vi "Process.vi"(8 "error in":errorcluster, 11 "Oxford1820 UI in":refnum<class "Instrument UI.Oxford1820.lvclass">) -> (0 "error out":errorcluster, 3 "Oxford1820 UI out":refnum<class "Instrument UI.Oxford1820.lvclass">)   [LabVIEW 2019, in "Instrument UI.Oxford1820.lvclass"]
doc: "---------------------------------------------------------------\nJKI State Machine Objects™\nhttp://jki.net/state-machine-objects/\nCopyright (C) 2005-2015, JKI <info@jki.net>\nALL RIGHTS RESERVEDJKI State Machine Objects (SMO) 1.0.0.5\nJKI - JKI\nCopyright (c) 2016, JKI"
uses:
  Instrument UI.Oxford1820.lvclass
  C:/Program Files/National Instruments/LabVIEW 2019/vi.lib/JKI/JKI SMO/SMO/SMO.lvclass
  C:/Program Files/National Instruments/LabVIEW 2019/user.lib/LevyLab/Instrument Framework/Instrument UI/Instrument UI.lvclass
  C:/Program Files/National Instruments/LabVIEW 2019/vi.lib/JKI/JKI SMO/SMO.UI/SMO.UI.lvclass
  <instrlib>/Mercury iXX/Public/Libraries/Magnet/Controls/Switch Heater.ctl
  Instrument.Oxford1820/Typedefs/getAll.ctl
  Instrument.Oxford1820/Instrument.Oxford1820.lvclass
  C:/Program Files/National Instruments/LabVIEW 2019/user.lib/LevyLab/Instrument Framework/Instrument/Instrument.lvclass
  <userlib>/LevyLab/Instrument Framework/Instrument UI/Instrument UI.lvclass/Instrument UI.ctl
  Instrument.Oxford1820/Instrument.Oxford1820.lvclass/Instrument.Oxford1820.ctl
  <vilib>/JKI/JKI SMO/SMO/SMO.lvclass/SMO.ctl
  <userlib>/LevyLab/Instrument Framework/Instrument/Typedefs/Client Type--Enum.ctl
  <userlib>/LevyLab/Instrument Framework/Instrument/Instrument.lvclass/Instrument.ctl
  Instrument.Oxford1820/Typedefs/Fill Mode-Combo.ctl
  <vilib>/JKI/JKI SMO/SMO/Private/ReftoDVR--SMO.vi
  <userlib>/LevyLab/Instrument Framework/Instrument/Instrument.lvclass
  <userlib>/LevyLab/Instrument Framework/Instrument UI/Instrument UI.lvclass
  <vilib>/JKI/JKI SMO/SMO/SMO.lvclass
  <vilib>/JKI/JKI SMO/SMO.UI/SMO.UI.lvclass
  <instrlib>/Mercury iXX/Public/Libraries/Magnet.lvlib
panel:
  in  "Clamp":bool
  in  "Open Target":dbl=100.0 format="%.1f (%%)"
  out "System Time (HH:MM:SS)":dbl=165.3592643737793 format="%<%I:%M:%S %p>T"
  out "LPF on":dbl format="%<%H:%M:%S>t"
  out "PS Heat on (HH:MM:SS)":dbl format="%<%H:%M:%S%1u>t"
  out "ETA":dbl=3660699600.0 format="%<%I:%M:%S %p %m/%d/%Y>T"
  out "version":string="v20/10/28"
  out "Level Graph":cluster{timestamp[], dbl[]}[](graph)
  out "N2 LEVEL":dbl format="%.0f %"
  in  "Window Maximize":bool
  in  "Window Minimize":bool
  out "Magnet Status 3":string="Status: Clamped"
  out "Voltage Meter":dbl(knob) caption="Voltage (V)" scale=-10.0..10.0
  out "Current Meter":dbl(knob) caption="Voltage (V)" scale=-180.0..180.0
  out "Magnet Field Meter":dbl(knob) caption="Voltage (V)" scale=-20.0..20.0
  in  "Hold":bool
  in  "To Set":bool
  in  "Send To IPS":bool
  out "PSU Field":dbl format="%#.5f T"
  in  "Target Field (T)":dbl caption="Field" format="%.2f"
  out "Target Field (T)":dbl caption="Field" format="%.2f T"
  in  "Target Rate (T/min)":dbl=0.1 caption="Rate" min=0.0 max=1.0 format="%.2f"
  out "Target Rate (T/min)":dbl caption="Rate" format="%.2f T/min"
  out "Field":dbl format="%.5f T"
  out "He LEVEL":dbl format="%.0f %"
  in  "PS Heat":bool
  in  "To Zero":bool
  out "N2 LVL":dbl format="%.1f (%%)"
  out "He LVL Chart":dbl(slide)=52.0833 scale=0.0..100.0
  out "N2 LVL Chart":dbl(slide)=61.3025 scale=0.0..100.0
  out "He LVL":dbl format="%.1f (%%)"
  in  "Fast/Slow Fill":bool
  in  "Open Needle Valve":bool
  in  "Close Needle Valve":bool
  in  "LPF Power":bool
  out "Needle Valve":dbl format="%.1f (%%)"
  out "Pressure":dbl format="%_5f mB"
  out "Magnet T":dbl format="%_2f K"
  out "Magnet R":dbl format="%_3f ohms"
  out "Voltage":dbl format="%.5f V"
  out "Current":dbl format="%.5f A"
  out "Magnet Status 2":string="Status: Clamped"
  # "Actions"
  # "Targets"
  # "Status"
  # "LPF"
  # "Needle Valve"
  # "IPS"
  # "PS Switch"
  # "Level"
  # "Level Graph"
  # "Rates"
  # "Slow Rates\nCurrent Range (A)     Field Range (T)  Rate (T/min)\n0       -- 100        0    -- 11.5     0.91\n100     -- 150        11.5 -- 17.2     0.23\n150     -- 155.467    17.2 -- 18       0.11\n155.567 -- 172.471    18   -- 20       0.11\nFast Rates\nCurrent Range (A)     Field Range (T)  Rate (T/min)\n0       -- 155.467    0    -- 18       1.0\n155.567 -- 172.471    18   -- 20       0.25"
  # "Helium"
  # "Nitrogen"
  # "Slow Rates\nCurrent Range (A)     Field Range (T)   Rate (T/min)\n0       -- 100        0    -- 11.5      0.91\n100     -- 150        11.5 -- 17.2      0.23\n150     -- 155.467    17.2 -- 18        0.11\n155.567 -- 172.471    18   -- 20        0.11\n\nFast Rates\nCurrent Range (A)     Field Range (T)   Rate (T/min)\n0       -- 155.467    0    -- 18        1.0\n155.567 -- 172.471    18   -- 20        0.25"
  # "SMO UI Template"
  # "For instructions on how to use the JKI State Machine Objects, examples and video tutorials, visit:\nhttp://jki.net/state-machine-objects/\n\nJKI State Machine Objects™\nhttp://jki.net/state-machine-objects/\nCopyright (C) 2005-2015, JKI <info@jki.net>\nALL RIGHTS RESERVED"
  # "Voltage (V)"
  # "Current (A)"
  # "Magnet (T)"
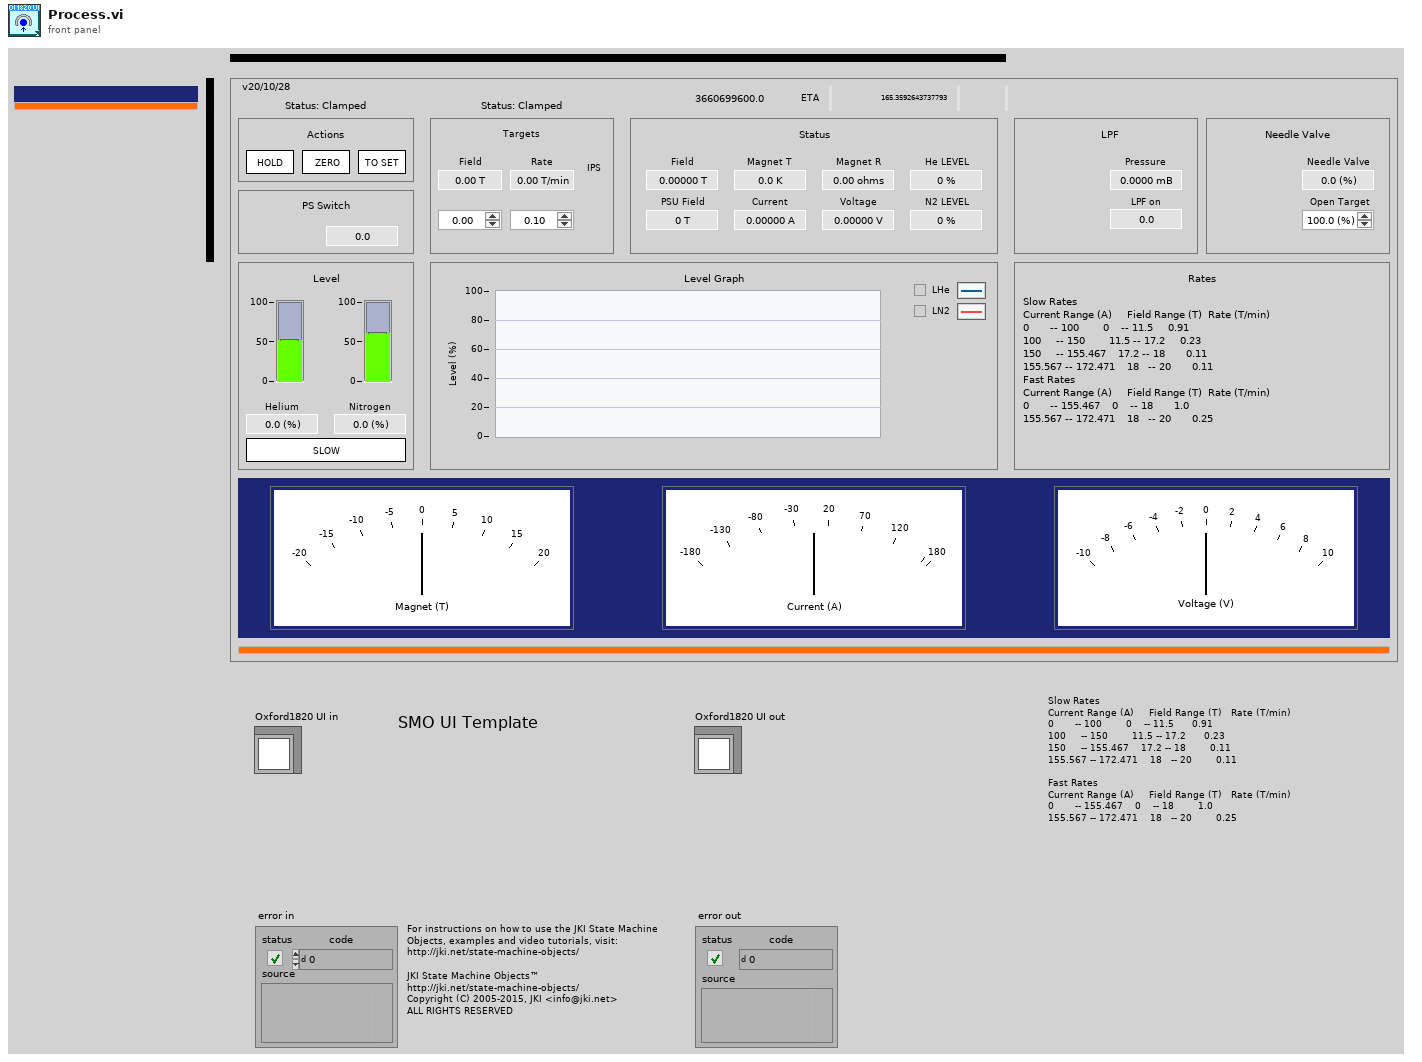
[diagram p1: front panel]
types:
  T1 = typedef "Mercury iXX.lvlib/Magnet.lvlib/Switch Heater.ctl" = string
  T2 = typedef "Instrument.Oxford1820.lvclass/getAll.ctl" = cluster{"1820_IPS_Magnet_Field":dbl, "1820_IPS_PS_Field":dbl, "1820_IPS_Target_Field":dbl, "1820_IPS_Target_Field_Rate":dbl, "1820_IPS_Voltage":dbl, "1820_IPS_Current":dbl, "1820_IPS_Level_N2":dbl, "1820_IPS_Level_He":dbl, "1820_IPS_Magnet_Temperature":dbl, "1820_IPS_Magnet_Temperature_R":dbl, "1820_IPS_M1_Current":dbl, "1820_IPS_M1_Voltage":dbl, "1820_IPS_M2_Current":dbl, "1820_IPS_M2_Voltage":dbl, "1820_IPS_M3_Current":dbl, "1820_IPS_M3_Voltage":dbl, "1820_IPS_Status":string, "1820_IPS_Switch":string, "1820_ITC_Lambda_Temperature":dbl, "1820_ITC_Lambda_Temperature_R":dbl, "1820_ITC_Pressure":dbl, "1820_ITC_Needle_Valve":dbl}
  T3 = enum32{"invalid app kind", "Development System", "Run Time System", "Student Edition", "Embedded LabVIEW", "Evaluation", "Custom"}
  T4 = enum32{"Invalid", "Standard", "Closed", "Hidden", "Minimized", "Maximized"}
  T5 = typedef "Instrument.lvlib/Instrument.lvclass/Client Type--Enum.ctl" = enum16{"Remote", "Local"}
  T6 = typedef "Instrument.Oxford1820.lvclass/Fill Mode-Combo.ctl" = string
  T7 = typedef "RemoteControl.lvlib/RemoteControl.lvclass/Message--Cluster.ctl" = cluster{"Command":string, "Data":variant, "ID":string, "error":errorcluster}
  T8 = cluster{"Core":cluster{"Current VI Reference":refnum<vi>, "Close Panel on Exit?":bool, "error":errorcluster}, "Instrument UI":refnum<class "Instrument UI.Oxford1820.lvclass">, "Instrument":refnum<class "Instrument.Oxford1820.lvclass">, "getAll":T2, "Response":string, "config":variant, "switch time on":timestamp, "switch time off":timestamp, "LPF time":timestamp}
  T9 = typedef "Instrument.Oxford1820.lvclass/PublicEvents--Instrument.Oxford1820.ProcessStatus.ctl" = string
  T10 = cluster{"Current VI Reference":refnum<vi>, "Close Panel on Exit?":bool, "error":errorcluster}
  T11 = typedef "LVRectTypeDef.ctl" = cluster{"Left":i16, "Top":i16, "Right":i16, "Bottom":i16}
  T12 = typedef "SMO.lvclass/Protected Events.ctl" = cluster{"StopProcesses":refnum<user-event>, "AbortProcesses":refnum<user-event>, "Config Changed":refnum<user-event>, "Dependency":refnum<user-event>}
  T13 = typedef "Instrument.lvlib/Instrument.lvclass/PublicEvents--Cluster.ctl" = cluster{"MessageFromProcess":refnum<user-event>}
  T14 = typedef "Instrument.Oxford1820.lvclass/PublicEvents--Cluster.ctl" = cluster{"ProcessStatus":refnum<user-event>}
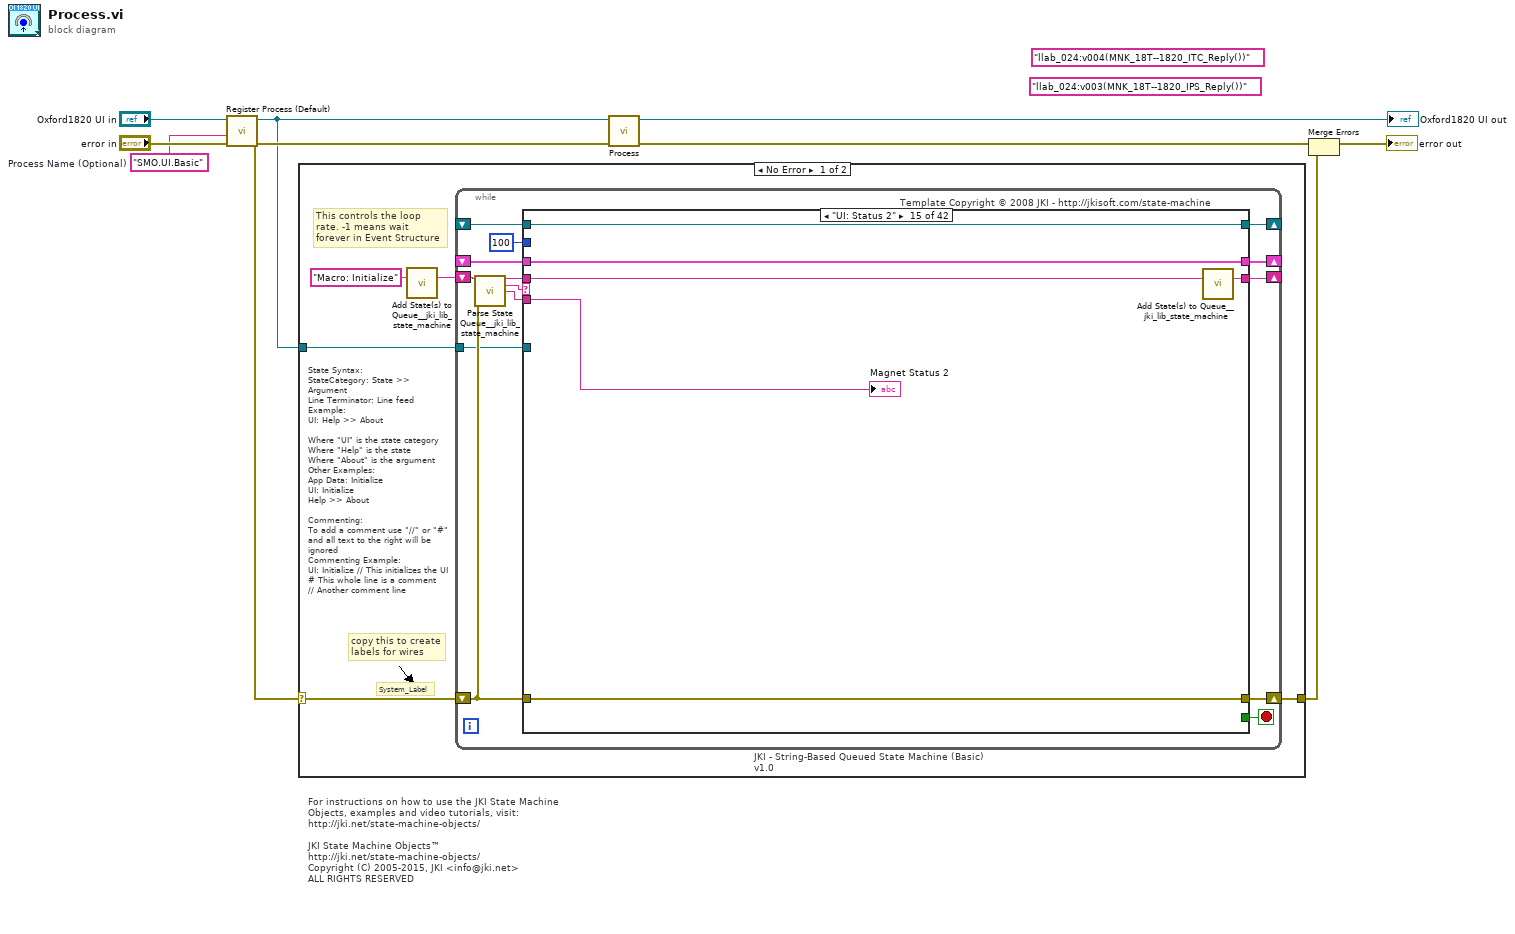
[diagram p0: block diagram]
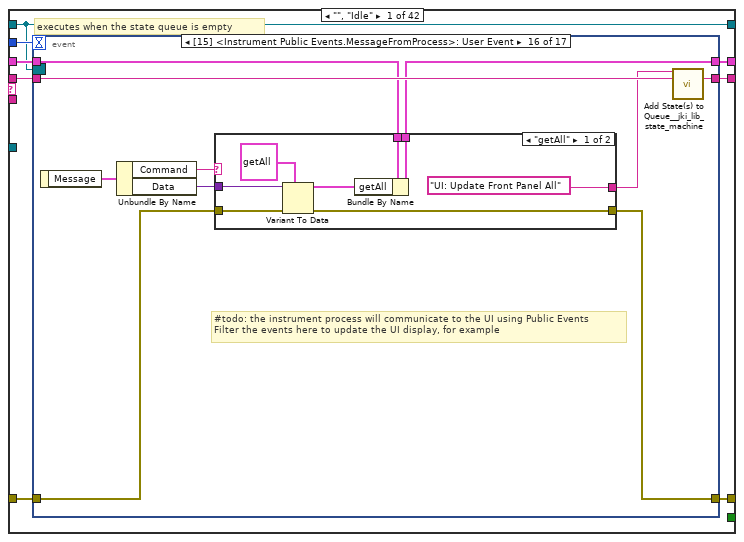
[diagram p2: hidden frame]
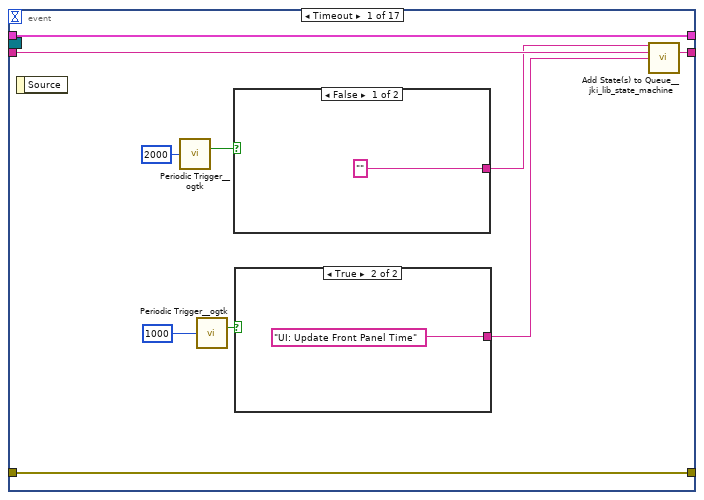
[diagram p3: hidden frame]
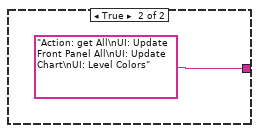
[diagram p4: hidden frame]
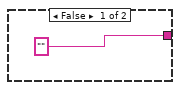
[diagram p5: hidden frame]
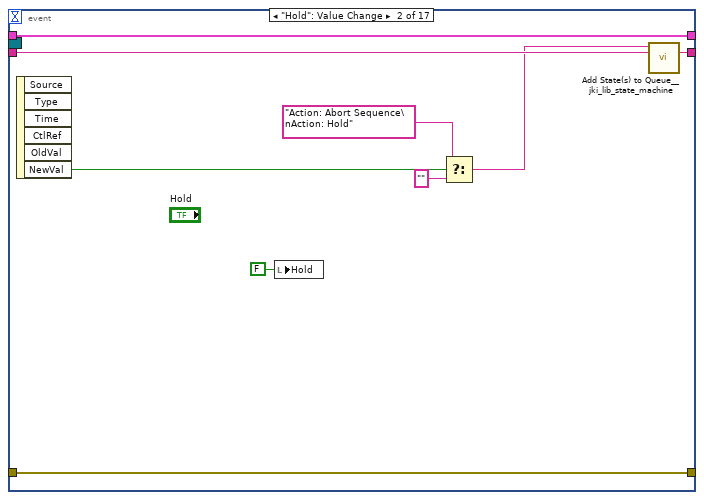
[diagram p6: hidden frame]
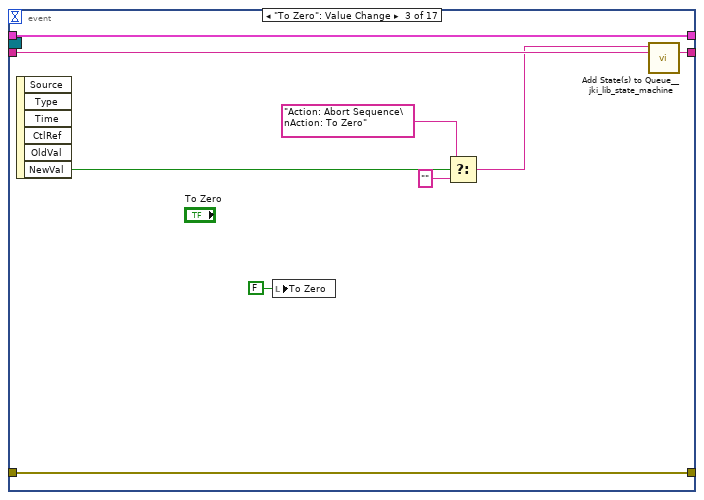
[diagram p7: hidden frame]
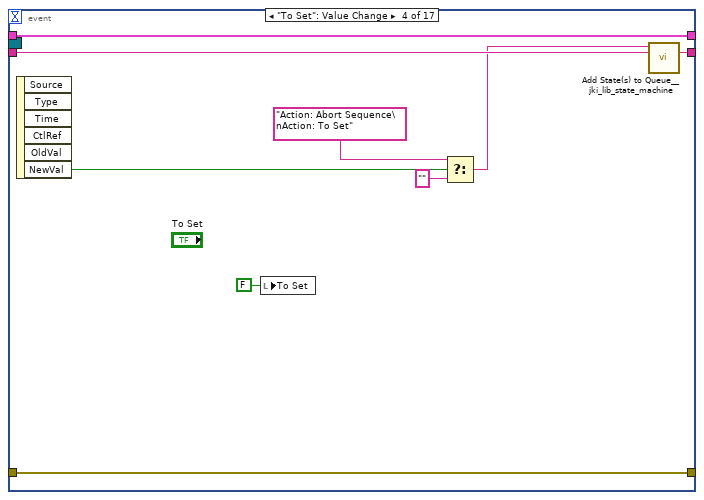
[diagram p8: hidden frame]
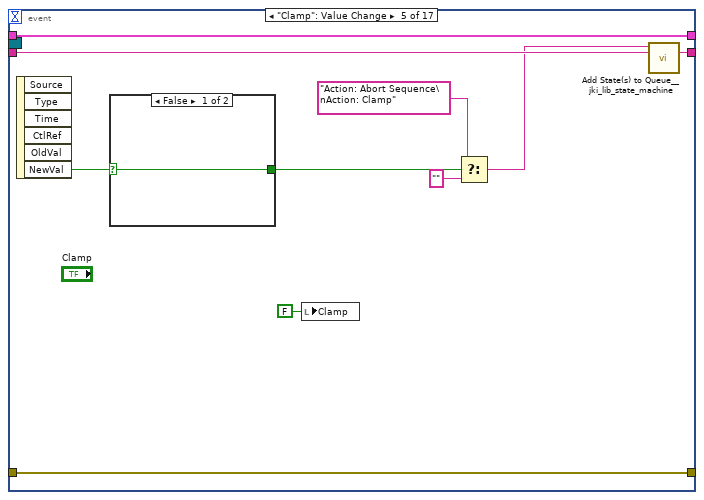
[diagram p9: hidden frame]
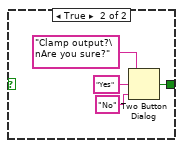
[diagram p10: hidden frame]
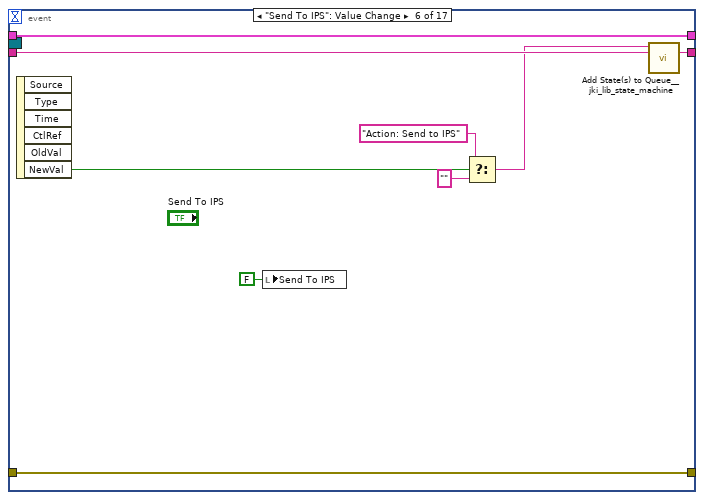
[diagram p11: hidden frame]
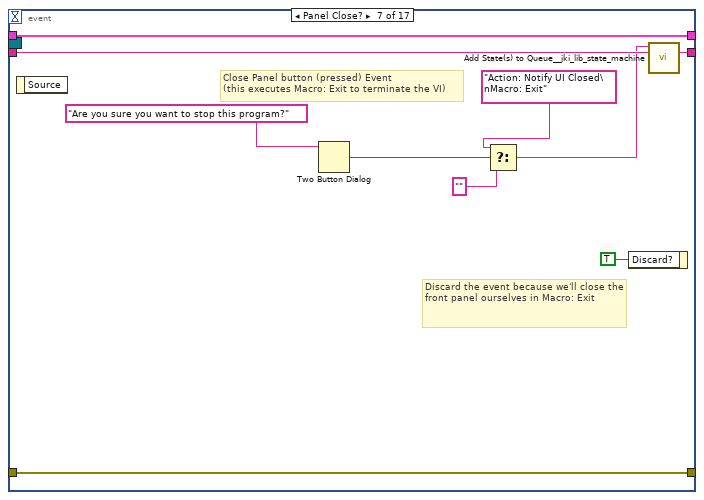
[diagram p12: hidden frame]
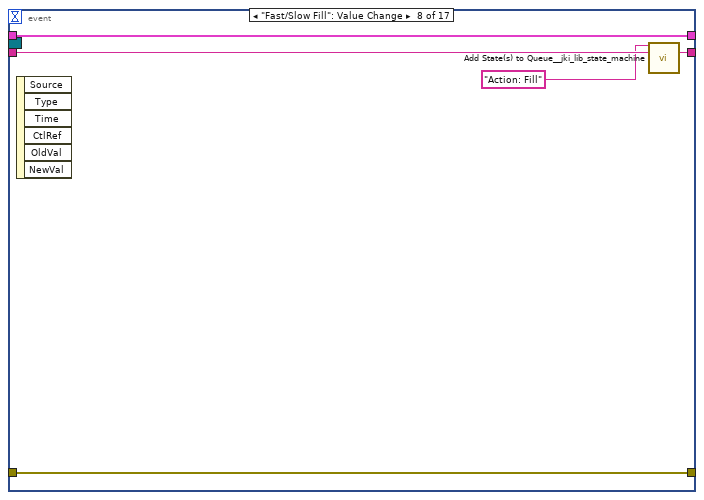
[diagram p13: hidden frame]
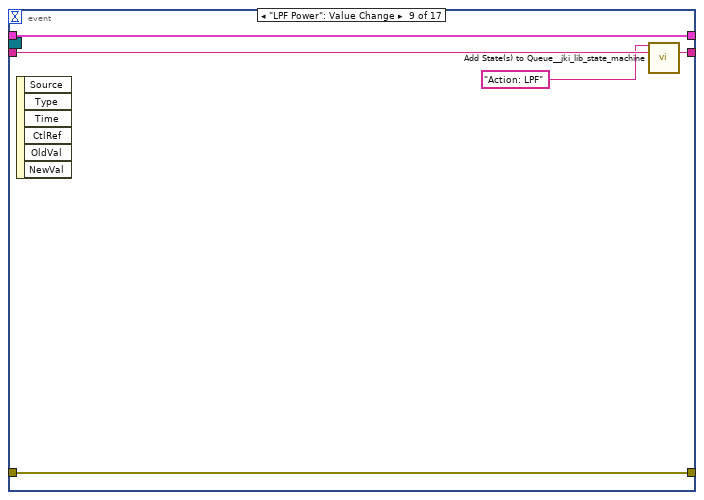
[diagram p14: hidden frame]
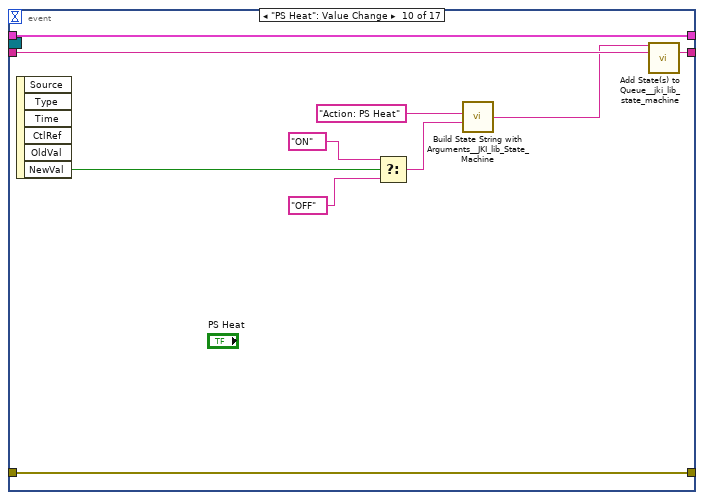
[diagram p15: hidden frame]
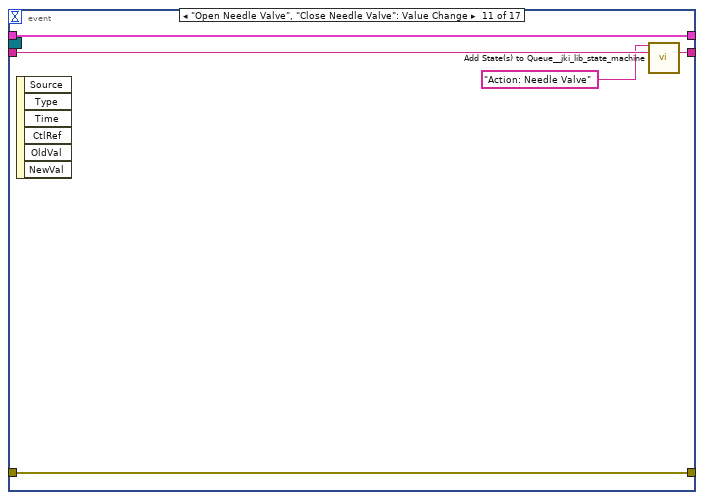
[diagram p16: hidden frame]
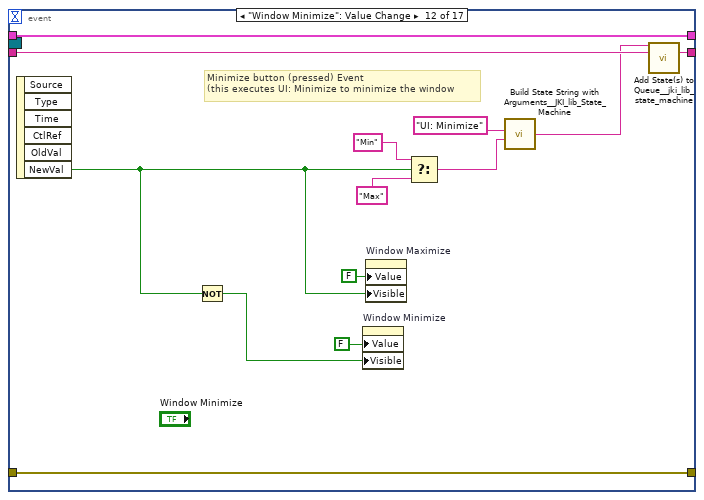
[diagram p17: hidden frame]
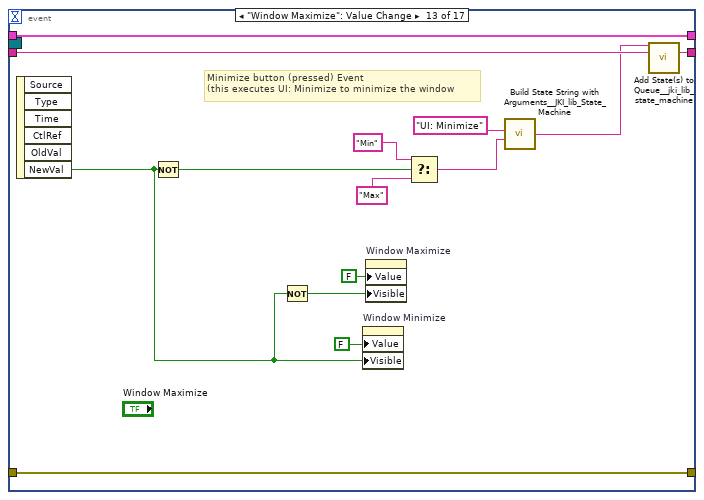
[diagram p18: hidden frame]
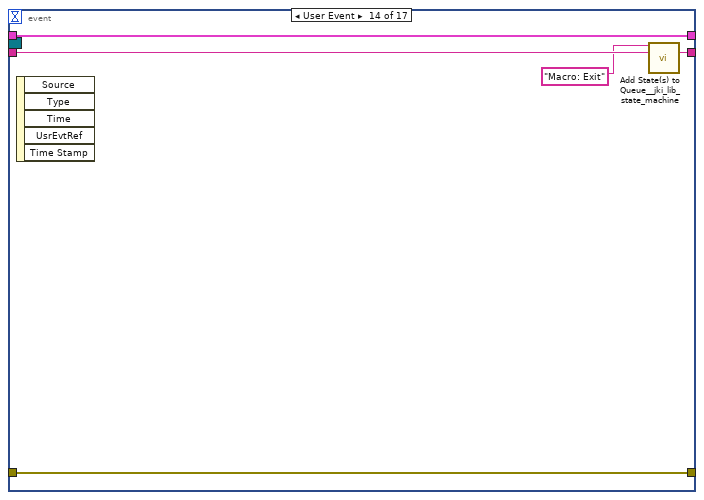
[diagram p19: hidden frame]
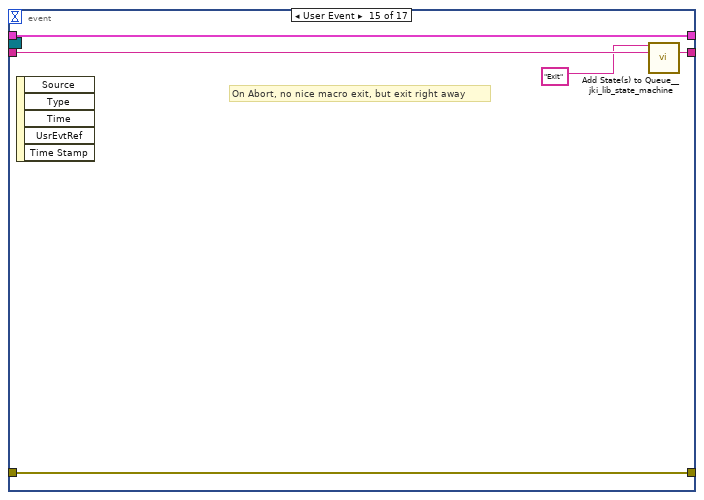
[diagram p20: hidden frame]
diagram:
  (unwired) "llab_024:v004(MNK_18T--1820_ITC_Reply())" ("variable")
  (unwired) "llab_024:v003(MNK_18T--1820_IPS_Reply())" ("variable")
  w1 = "SMO.UI.Basic"  # Process Name (Optional)
  # "For instructions on how to use the JKI State Machine Objects, examples and video tutorials, visit:\nhttp://jki.net/state-machine-objects/\n\nJKI State Machine Objects™\nhttp://jki.net/state-machine-objects/\nCopyright (C) 2005-2015, JKI <info@jki.net>\nALL RIGHTS RESERVED"
  n1 = call <vilib>:"Register Process (Default).vi"("error in (no error)"="error in", "Process Name (optional)"=w1, "SMO"="Oxford1820 UI in") -> ("error out"=w6:errorcluster, "SelfRef"=w5:refnum<class "Instrument UI.Oxford1820.lvclass">)  [unwired: 7 in]
  n2 = case shown="No Error" w6 {
    selector: w6 -> [w11 w700]
    tunnel: w5 -> [w12 _]
    tunnel: [w10 w700] -> w2
    frame No Error {
      # "State Syntax:\nStateCategory: State >> Argument\nLine Terminator: Line feed\nExample:\nUI: Help >> About\n\nWhere \"UI\" is the state category\nWhere \"Help\" is the state\nWhere \"About\" is the argument\nOther Examples:\nApp Data: Initialize\nUI: Initialize\nHelp >> About\n\nCommenting:\nTo add a comment use \"//\" or \"#\" and all text to the right will be ignored\nCommenting Example:\nUI: Initialize // This initializes the UI\n# This whole line is a comment\n// Another comment line"
      # "copy this to create labels for wires"
      # "This controls the loop rate. -1 means wait forever in Event Structure"
      # "System_Label"
      n3 = call <vilib>:"Add State(s) to Queue__jki_lib_state_machine.vi"("State(s) in (\"\")"="Macro: Initialize") -> ("States Out"=w14:string)  [unwired: 14 in]
      n4 = while "JKI - String-Based Queued State Machine (Basic) v1.0" {
        shift-right: [w15] -> _
        shift-left: _ -> [w21]
        shift-right: [w24] -> w10
        shift-left: w11 -> [w19]
        shift-right: [w23] -> _
        shift-left: w14 -> [w25]
        tunnel: w12 -> [w18]
        shift-right: [w17] -> _
        shift-left: _ -> [w16]
        stop <- w22 stop-if-true
        # "Template Copyright © 2008 JKI - http://jkisoft.com/state-machine"
        n5 = call <vilib>:"Parse State Queue__jki_lib_state_machine.vi"("State Queue"=w25, "Error In (no error)"=w19) -> ("Remaining States"=w27:string, "Current State"=w28:string, "Arguments"=w26:string)  [unwired: 11 in]
        n6 = case shown="\"UI: Status 2\"" w28 {
          selector: w28 -> [_ _ w215 _ _ _ _ _ _ _ _ _ _ _ _ _ _ _ _ _ _ _ _ _ _ _ _ _ _ _ _ _ _ _ _ _ _ _ _ _ _ _]
          tunnel: w27 -> [w36 w213 w219 w238 w252 w258 w263 w283 w290 w295 w310 w334 w362 w384 w390 w397 w404 w420 w454 w480 w489 w503 w508 w519 w526 w531 w547 w553 w560 w567 w577 w587 w596 w603 w612 w621 w630 w643 w657 w672 w688 w699]
          tunnel: w26 -> [_ _ _ _ _ _ _ _ _ _ _ _ _ _ w385 _ w398 w414 w455 _ _ _ _ _ _ _ _ _ _ _ _ _ _ _ _ _ _ _ _ _ w680 _]
          tunnel: w21 -> [w34 w210 w217 w229 w240 w254 w260 _ w285 w292 w308 w315 w359 w380 w387 w394 w402 w416 w453 w477 w485 w494 w505 w516 w521 w528 w545 w551 w556 w561 w574 w580 w588 w597 w606 w615 w624 w635 w648 w661 w679 w691]
          tunnel: [w33 w211 w221 w235 w245 w253 w261 w268 w286 w293 w305 w317 w354 w382 w388 w395 w399 w417 w448 w478 w487 w501 w506 w510 w522 w529 w542 w548 w557 w562 w572 w582 w593 w598 w609 w618 w627 w638 w652 w662 w684 w694] -> w24
          tunnel: w19 -> [w32 w211 w220 w235 w241 _ w261 w266 w287 w293 w306 w317 w354 w382 w388 w395 w400 w418 w449 w478 w487 w501 w506 w511 w523 w529 w533 w549 w557 w563 w569 w579 w591 w599 w607 w616 w625 w639 w653 w668 w685 w695]
          tunnel: [w35 w212 w218 w237 w251 w257 w262 w282 w289 w294 w309 w333 w361 w383 w389 w396 w403 w419 w459 w479 w488 w502 w507 w518 w525 w530 w546 w552 w559 w566 w576 w586 w595 w602 w611 w620 w629 w642 w656 w671 w687 w698] -> w23
          tunnel: [_ _ _ _ _ TRUE _ _ _ _ _ _ _ _ _ _ _ _ _ _ _ _ _ _ _ _ _ _ _ _ _ _ _ _ _ _ _ _ _ _ _ _] -> w22
          tunnel: 100 ("Timeout") -> [w30 _ _ _ _ _ _ _ _ _ _ _ _ _ _ _ _ _ _ _ _ _ _ _ _ _ _ _ _ _ _ _ _ _ _ _ _ _ _ _ _ _]
          tunnel: w18 -> [_ _ _ _ _ _ _ w267 _ _ _ _ _ _ _ _ _ _ _ _ _ _ _ _ _ _ _ _ _ _ _ _ _ _ _ _ _ _ _ _ _ _]
          tunnel: [w29 w209 w214 w226 w250 w255 w259 w280 w284 w291 w307 w332 w360 w381 w386 w393 w401 w413 w458 w476 w486 w495 w504 w517 w524 w527 w544 w550 w558 w565 w575 w585 w594 w601 w610 w619 w628 w641 w655 w670 w686 w697] -> w17
          tunnel: w16 -> [w29 w209 w214 w226 w250 w255 w259 w280 w284 w291 w307 w332 w360 w381 w386 w393 w401 w413 w458 w476 w486 w495 w504 w517 w524 w527 _ w550 w558 w565 w575 w585 w594 w601 w610 w619 w628 w641 w655 w670 w686 w697]
          tunnel: [w31 w210 w217 w236 w243 w254 w260 w281 w285 w292 w308 w316 w359 w380 w387 w394 w402 w416 w453 w477 w485 w494 w505 w516 w521 w528 w545 w551 w555 w561 w573 w584 w590 w597 w605 w614 w623 w634 w646 w660 w682 w690] -> w15
          frame "", "Idle" {
            # "executes when the state queue is empty"
            n7 = event shown="[15] <Instrument Public Events.MessageFromProcess>: User Event" {
              selector: w29 -> [_ _ _ _ _ _ _ _ _ _ _ _ _ _ _ _ _]
              dyn-events: _ -> [_ _ _ _ _ _ _ _ _ _ _ _ _ _ _ _ _]
              timeout: w30 -> [_ _ _ _ _ _ _ _ _ _ _ _ _ _ _ _ _]
              tunnel: w36 -> [w46 w59 w68 w77 w87 w101 w111 w116 w121 w131 w136 w149 w163 w168 w173 w183 w208]
              tunnel: [w45 w58 w67 w76 w86 w100 w110 w115 w120 w130 w135 w148 w162 w167 w172 w182 w207] -> w35
              tunnel: w34 -> [w42 w56 w65 w74 w84 w98 w108 w114 w119 w129 w134 w147 w161 w165 w170 w181 w201]
              tunnel: [w44 w57 w66 w75 w85 w99 w107 w113 w118 w128 w133 w146 w160 w166 w171 w174 w205] -> w33
              tunnel: w32 -> [w44 w57 w66 w75 w85 w99 w107 w113 w118 w128 w133 w146 w160 w166 w171 w175 w202]
              tunnel: [w42 w56 w65 w74 w84 w98 w108 w114 w119 w129 w134 w147 w161 w165 w170 w180 w201] -> w31
              event Timeout {
                n8 = event-data() -> ()  [unwired: 1 in, 1 out]
                n9 = call <userlib>:"Periodic Trigger__ogtk.vi"("time (ms)"=u32 2000 ("update time (ms)")) -> ("Triggered"=w38:bool)  [unwired: 12 in, 2 out]
                n10 = call <userlib>:"Periodic Trigger__ogtk.vi"("time (ms)"=u32 1000 ("update time (ms)")) -> ("Triggered"=w40:bool)  [unwired: 12 in, 2 out]
                n11 = case shown="False" w38 {
                  tunnel: ["" "Action: get All\nUI: Update Front Panel All\nUI: Update Chart\nUI: Level Colors"] -> w43
                  frame False {
                  }
                  frame True {
                  }
                }
                n12 = case shown="True" w40 {
                  tunnel: ["" "UI: Update Front Panel Time"] -> w39
                  frame False {
                  }
                  frame True {
                  }
                }
                n13 = call <vilib>:"Add State(s) to Queue__jki_lib_state_machine.vi"("State(s) in Front (\"\")"=w43, "State(s) in (\"\")"=w46, "State(s) at Back (\"\")"=w39) -> ("States Out"=w45:string)  [unwired: 12 in]
              }
              event "Hold": Value Change {
                n14 = event-data() -> ("NewVal"=w55:bool)  [unwired: 1 in, 5 out]
                n15 = local write "Hold"(FALSE ("Hold")) -> ()
                n16 = Select(t="Action: Abort Sequence\nAction: Hold" ("State(s) in Front (\"\")"), s=w55, f="") -> (s? t:f=w52:string)
                n17 = call <vilib>:"Add State(s) to Queue__jki_lib_state_machine.vi"("State(s) in Front (\"\")"=w52, "State(s) in (\"\")"=w59) -> ("States Out"=w58:string)  [unwired: 13 in]
              }
              event "To Zero": Value Change {
                n18 = event-data() -> ("NewVal"=w63:bool)  [unwired: 1 in, 5 out]
                n19 = local write "To Zero"(FALSE ("To Zero")) -> ()
                n20 = Select(t="Action: Abort Sequence\nAction: To Zero" ("State(s) in Front (\"\")"), s=w63, f="") -> (s? t:f=w61:string)
                n21 = call <vilib>:"Add State(s) to Queue__jki_lib_state_machine.vi"("State(s) in Front (\"\")"=w61, "State(s) in (\"\")"=w68) -> ("States Out"=w67:string)  [unwired: 13 in]
              }
              event "To Set": Value Change {
                n22 = event-data() -> ("NewVal"=w72:bool)  [unwired: 1 in, 5 out]
                n23 = local write "To Set"(FALSE ("To Set")) -> ()
                n24 = Select(t="Action: Abort Sequence\nAction: To Set" ("State(s) in Front (\"\")"), s=w72, f="") -> (s? t:f=w70:string)
                n25 = call <vilib>:"Add State(s) to Queue__jki_lib_state_machine.vi"("State(s) in Front (\"\")"=w70, "State(s) in (\"\")"=w77) -> ("States Out"=w76:string)  [unwired: 13 in]
              }
              event "Clamp": Value Change {
                n26 = event-data() -> ("NewVal"=w78:bool)  [unwired: 1 in, 5 out]
                n27 = case shown="False" w78 {
                  selector: w78 -> [w88 _]
                  tunnel: [w88 w89] -> w79
                  frame False {
                  }
                  frame True {
                    n28 = Two Button Dialog(message="Clamp output?\nAre you sure?", 1:"No" ("F button name (\"Cancel\")"), 2:"Yes" ("T button name (\"OK\")")) -> (T button?=w89:bool)
                  }
                }
                n29 = local write "Clamp"(FALSE ("Clamp")) -> ()
                n30 = Select(t="Action: Abort Sequence\nAction: Clamp" ("State(s) in Front (\"\")"), s=w79, f="") -> (s? t:f=w81:string)
                n31 = call <vilib>:"Add State(s) to Queue__jki_lib_state_machine.vi"("State(s) in Front (\"\")"=w81, "State(s) in (\"\")"=w87) -> ("States Out"=w86:string)  [unwired: 13 in]
              }
              event "Send To IPS": Value Change {
                n32 = event-data() -> ("NewVal"=w97:bool)  [unwired: 1 in, 5 out]
                n33 = local write "Send To IPS"(FALSE ("Send to IPS")) -> ()
                n34 = Select(t="Action: Send to IPS" ("State(s) in Front (\"\")"), s=w97, f="") -> (s? t:f=w94:string)
                n35 = call <vilib>:"Add State(s) to Queue__jki_lib_state_machine.vi"("State(s) in Front (\"\")"=w94, "State(s) in (\"\")"=w101) -> ("States Out"=w100:string)  [unwired: 13 in]
              }
              event Panel Close? {
                # "Discard the event because we'll close the front panel ourselves in Macro: Exit"
                # "Close Panel button (pressed) Event\n(this executes Macro: Exit to terminate the VI)"
                n36 = event-data() -> ()  [unwired: 1 in, 1 out]
                n37 = Two Button Dialog(message="Are you sure you want to stop this program?") -> (T button?=w106:bool)  [unwired: 2 in]
                n38 = Select(t="Action: Notify UI Closed\nMacro: Exit", s=w106, f="") -> (s? t:f=w102:string)
                n39 = event-data("Discard?"=TRUE) -> ()  [unwired: 1 in, 1 out]
                n40 = call <vilib>:"Add State(s) to Queue__jki_lib_state_machine.vi"("State(s) in Front (\"\")"=w102, "State(s) in (\"\")"=w111) -> ("States Out"=w110:string)  [unwired: 13 in]
              }
              event "Fast/Slow Fill": Value Change {
                n41 = event-data() -> ()  [unwired: 1 in, 6 out]
                n42 = call <vilib>:"Add State(s) to Queue__jki_lib_state_machine.vi"("State(s) in Front (\"\")"="Action: Fill", "State(s) in (\"\")"=w116) -> ("States Out"=w115:string)  [unwired: 13 in]
              }
              event "LPF Power": Value Change {
                n43 = event-data() -> ()  [unwired: 1 in, 6 out]
                n44 = call <vilib>:"Add State(s) to Queue__jki_lib_state_machine.vi"("State(s) in Front (\"\")"="Action: LPF", "State(s) in (\"\")"=w121) -> ("States Out"=w120:string)  [unwired: 13 in]
              }
              event "PS Heat": Value Change {
                n45 = event-data() -> ("NewVal"=w122:bool)  [unwired: 1 in, 5 out]
                n46 = Select(t=T1 "ON" ("LPF State"), s=w122, f=T1 "OFF" ("LPF State")) -> (s? t:f=w124:T1)
                n47 = call <vilib>:"Build State String with Arguments__JKI_lib_State_Machine.vi"("Arguments (\"\")"=w124, "State"="Action: PS Heat") -> ("State with Arguments"=w123:string)  [unwired: 4 in]
                n48 = call <vilib>:"Add State(s) to Queue__jki_lib_state_machine.vi"("State(s) in Front (\"\")"=w123, "State(s) in (\"\")"=w131) -> ("States Out"=w130:string)  [unwired: 13 in]
              }
              event "Open Needle Valve", "Close Needle Valve": Value Change {
                n49 = event-data() -> ()  [unwired: 1 in, 6 out]
                n50 = call <vilib>:"Add State(s) to Queue__jki_lib_state_machine.vi"("State(s) in Front (\"\")"="Action: Needle Valve", "State(s) in (\"\")"=w136) -> ("States Out"=w135:string)  [unwired: 13 in]
              }
              event "Window Minimize": Value Change {
                # "Minimize button (pressed) Event\n(this executes UI: Minimize to minimize the window"
                n51 = event-data() -> ("NewVal"=w137:bool)  [unwired: 1 in, 5 out]
                n52 = Not(x=w137) -> (.not. x?=w138:bool)
                n53 = property on="Window Minimize" class="Bool (strict)"("Value"=FALSE ("Window Maximize"), "Visible"=w138) -> ()  [unwired: 2 in, 2 out]
                n54 = property on="Window Maximize" class="Bool (strict)"("Value"=FALSE ("Window Maximize"), "Visible"=w137) -> ()  [unwired: 2 in, 2 out]
                n55 = Select(t="Min" ("Arguments (\"\")"), s=w137, f="Max" ("Arguments (\"\")")) -> (s? t:f=w142:string)
                n56 = call <vilib>:"Build State String with Arguments__JKI_lib_State_Machine.vi"("Arguments (\"\")"=w142, "State"="UI: Minimize") -> ("State with Arguments"=w141:string)  [unwired: 4 in]
                n57 = call <vilib>:"Add State(s) to Queue__jki_lib_state_machine.vi"("State(s) in Front (\"\")"=w141, "State(s) in (\"\")"=w149) -> ("States Out"=w148:string)  [unwired: 13 in]
              }
              event "Window Maximize": Value Change {
                # "Minimize button (pressed) Event\n(this executes UI: Minimize to minimize the window"
                n58 = event-data() -> ("NewVal"=w151:bool)  [unwired: 1 in, 5 out]
                n59 = Not(x=w151) -> (.not. x?=w152:bool)
                n60 = Not(x=w151) -> (.not. x?=w150:bool)
                n61 = property on="Window Minimize" class="Bool (strict)"("Value"=FALSE ("Window Maximize"), "Visible"=w151) -> ()  [unwired: 2 in, 2 out]
                n62 = property on="Window Maximize" class="Bool (strict)"("Value"=FALSE ("Window Maximize"), "Visible"=w150) -> ()  [unwired: 2 in, 2 out]
                n63 = Select(t="Min" ("Arguments (\"\")"), s=w152, f="Max" ("Arguments (\"\")")) -> (s? t:f=w156:string)
                n64 = call <vilib>:"Build State String with Arguments__JKI_lib_State_Machine.vi"("Arguments (\"\")"=w156, "State"="UI: Minimize") -> ("State with Arguments"=w155:string)  [unwired: 4 in]
                n65 = call <vilib>:"Add State(s) to Queue__jki_lib_state_machine.vi"("State(s) in Front (\"\")"=w155, "State(s) in (\"\")"=w163) -> ("States Out"=w162:string)  [unwired: 13 in]
              }
              event User Event {
                n66 = event-data() -> ()  [unwired: 1 in, 5 out]
                n67 = call <vilib>:"Add State(s) to Queue__jki_lib_state_machine.vi"("State(s) in Front (\"\")"="Macro: Exit", "State(s) in (\"\")"=w168) -> ("States Out"=w167:string)  [unwired: 13 in]
              }
              event User Event {
                # "On Abort, no nice macro exit, but exit right away"
                n68 = event-data() -> ()  [unwired: 1 in, 5 out]
                n69 = call <vilib>:"Add State(s) to Queue__jki_lib_state_machine.vi"("State(s) in Front (\"\")"="Exit", "State(s) in (\"\")"=w173) -> ("States Out"=w172:string)  [unwired: 13 in]
              }
              event User Event {
                # "#todo: the instrument process will communicate to the UI using Public Events\nFilter the events here to update the UI display, for example"
                n70 = event-data() -> ("Message"=w176:T7)  [unwired: 1 in]
                n71 = Unbundle By Name(w176) -> ("Command"=w178:string, "Data"=w179:variant)
                n72 = case shown="\"getAll\"" w178 {
                  tunnel: w179 -> [w188 w199]
                  tunnel: w181 -> [w191 w200]
                  tunnel: [w190 w200] -> w180
                  tunnel: ["UI: Update Front Panel All" w196] -> w177
                  tunnel: w175 -> [w185 w193]
                  tunnel: [w184 w192] -> w174
                  frame "getAll" {
                    n73 = Variant To Data(error in=w185, type=T2 {"1820_IPS_Magnet_Field"=0.0, "1820_IPS_PS_Field"=0.0, "1820_IPS_Target_Field"=0.0, "1820_IPS_Target_Field_Rate"=0.0, "1820_IPS_Voltage"=0.0, "1820_IPS_Current"=0.0, "1820_IPS_Level_N2"=0.0, "1820_IPS_Level_He"=0.0, "1820_IPS_Magnet_Temperature"=0.0, "1820_IPS_Magnet_Temperature_R"=0.0, "1820_IPS_M1_Current"=0.0, "1820_IPS_M1_Voltage"=0.0, "1820_IPS_M2_Current"=0.0, "1820_IPS_M2_Voltage"=0.0, "1820_IPS_M3_Current"=0.0, "1820_IPS_M3_Voltage"=0.0, "1820_IPS_Status"="", "1820_IPS_Switch"="", "1820_ITC_Lambda_Temperature"=0.0, "1820_ITC_Lambda_Temperature_R"=0.0, "1820_ITC_Pressure"=0.0, "1820_ITC_Needle_Valve"=0.0} ("getAll"), Variant=w188) -> (data=w186:T2, error out=w184:errorcluster)
                    n74 = Bundle By Name(cluster=w191, "getAll"=w186) -> (w190:T8)
                  }
                  frame Default {
                    n75 = Variant To Data(error in=w193, type="", Variant=w199) -> (data=w195:string, error out=w194:errorcluster)
                    n76 = Format Into String(format string="UI: Status 2 >> %s", error in=w194, w195) -> (resulting string=w196:string, error out=w192:errorcluster)  [unwired: 1 in]
                  }
                }
                n77 = call <vilib>:"Add State(s) to Queue__jki_lib_state_machine.vi"("State(s) in Front (\"\")"=w177, "State(s) in (\"\")"=w183) -> ("States Out"=w182:string)  [unwired: 13 in]
              }
              event User Event {
                # "#todo: the instrument process will communicate to the UI using Public Events\nFilter the events here to update the UI display, for example"
                n78 = event-data() -> ("ProcessStatus"=w203:T9)  [unwired: 1 in]
                n79 = Format Into String(format string="UI: Status 2 >> %s", error in=w202, w203) -> (resulting string=w206:string, error out=w205:errorcluster)  [unwired: 1 in]
                n80 = call <vilib>:"Add State(s) to Queue__jki_lib_state_machine.vi"("State(s) in Front (\"\")"=w206, "State(s) in (\"\")"=w208) -> ("States Out"=w207:string)  [unwired: 13 in]
              }
            }
          }
          frame "---------- Core ----------" {
            # "Do not put any code in this frame.\n(it is a separator no-op)"
            n81 = call <vilib>:"Add State(s) to Queue__jki_lib_state_machine.vi"("State(s) in (\"\")"=w213) -> ("States Out"=w212:string)  [unwired: 14 in]
          }
          frame Default {
            w224 = 42 items=["No error", "Argument error", "Memory is full", "Out of zone", "End of file", "File already open", "Generic file I/O error", "File not found", "File permission error", "Disk is full", "Duplicate path", "Too many files open", "System feature not enabled", "Resource file not found", "Cannot add resource", "Resource not found", "Image not found", "Image memory error", "Pen does not exist", "Config type invalid", "Config token not found", "Config parse error", "Config memory error", "Bad external code format", "Bad external code offset", "External code not present", "Null window", "Destroy window error", "Null menu", "Print aborted", "Bad print record", "Print driver error", "Windows error during printing", "Memory error during printing", "Print dialog error", "Generic print error", "Invalid device refnum", "Device not found", "Device parameter error", "Device unit error", "Cannot open device", "Device call aborted", "Generic error", "Cancelled by user", "Object ID too low", "Object ID too high", "Object not in heap", "Unknown heap", "Unknown object (invalid DefProc)", "Unknown object (DefProc not in table)", "Message out of range", "Invalid (null) method", "Unknown message", "Manager call not supported", "Bad address", "Network operation in progress", "Network operation timed out", "Connection is busy", "Network attribute not supported", "Network error", "Address in use", "System out of memory", "Connection aborted", "Connection refused", "Not connected", "Already connected", "Connection closed", "Initialization error (interapplication manager)", "Bad occurrence", "Wait on unbound occurrence handler", "Occurrence queue overflow", "Datalog type conflict", "Unused", "Unrecognized type (interapplication manager)", "Memory corrupt", "Failed to make temporary DLL", "Old CIN version", "Drag socket not found", "Failed to load drop-object", "Failed to register OLE object", "Failed to release OLE object", "Format specifier type mismatch", "Unknown format specifier", "Too few format specifiers", "Too many format specifiers", "Scan failed", "Newer CIN version", "Error converting to variant", "Runtime menu error", "Password tampered", "Variant attribute not found", "Incompatible variant data type", "Event data is not available", "Event Store is not present", "Occurrence is not found", "Event Queue is not created", "Event info is not available", "Refnum passed is NULL", "Error retrieving Class GUID", "Error retrieving CoClass GUID", "Error retrieving TypeLib GUID.", "Bad built application magic bytes.", "Specific driver is different from the specific driver associated with the Logical Name.", "There is no session opened to the class driver.", "Max Error", "MAX - Error with config objects", "MAX - Error loading configuration", "MAX - Group not supported"]
            # "Current State"
            # "Do not delete, rename, or modify this frame.\n(this is used to capture unhandled states and typos)"
            # "Handle mistyped state name (developer tool)"
            n82 = Format Into String(format string="Software Exception: Unhandled State \"%s\"." ("message"), error in=w220, w215) -> (resulting string=w223:string, error out=w222:errorcluster)  [unwired: 1 in]
            n83 = call <vilib>:"Error Cluster From Error Code.vi"("show call chain? (False)"=TRUE, "error in (no error)"=w222, "error message (\"\")"=w223, "error code (0)"=w224) -> ("error out"=w221:errorcluster)  [unwired: 5 in]
            n84 = call <vilib>:"Add State(s) to Queue__jki_lib_state_machine.vi"("State(s) in (\"\")"=w219) -> ("States Out"=w218:string)  [unwired: 14 in]
          }
          frame "Initialize Core Data" {
            # "Do not delete, rename, or modify this frame.\n(this is used to determine panel behavior on exit)"
            # "originally closed?"
            # "exe?"
            # "If panel starts closed or is an EXE, then close it when we exit"
            n85 = property class="VI"() -> ("Front Panel.Open"=w234:bool)  [unwired: 2 in, 2 out]
            n86 = property class="App"() -> ("App.Kind"=w233:T3)  [unwired: 2 in, 2 out]
            n87 = control-ref of="Current VI Reference"() -> (w227:refnum<vi>)
            n88 = Not(x=w234) -> (.not. x?=w231:bool)
            n89 = Equal?(x=w233, y=T3."Run Time System" ("Application:Kind")) -> (x = y?=w230:bool)
            n90 = Or(x=w231, y=w230) -> (x .or. y?=w228:bool)
            n91 = Bundle By Name(cluster=w229, "Core.Current VI Reference"=w227, "Core.Close Panel on Exit?"=w228) -> (w236:T8)
            n92 = call <vilib>:"Add State(s) to Queue__jki_lib_state_machine.vi"("State(s) in (\"\")"=w238) -> ("States Out"=w237:string)  [unwired: 14 in]
          }
          frame "Error Handler" {
            w245 = errorcluster {"status"=FALSE, "code"=0, "source"=""}  # No error
            # "Overwrite this method to handle errors and pass to parent if not handled. Parent will fire a public event if the error is not handled up the chain of classes."
            # "Handle any errors here.\nYou can also output any states to clean-up after errors occur"
            n93 = Unbundle By Name(w240) -> ("Instrument UI"=w249:refnum<class "Instrument UI.Oxford1820.lvclass">)
            n94 = call-dynamic "Handle Error.vi"("Stop on Unhandled Error (T)"=FALSE, "error in"=w241, "SMO"=w249) -> ("handling error"=w239:errorcluster, "Unhandled error"=w244:errorcluster)  [unwired: 6 in, 1 out]
            n95 = Bundle By Name(cluster=w240, "Core.error"=w244) -> (w243:T8)
            n96 = Select(t="Exit", s=w239, f="") -> (s? t:f=w246:string)
            n97 = call <vilib>:"Add State(s) to Queue__jki_lib_state_machine.vi"("State(s) in Front (\"\")"=w246, "State(s) in (\"\")"=w252) -> ("States Out"=w251:string)  [unwired: 13 in]
          }
          frame "Exit" {
            # "Do not put any code in this frame.\n(No errors that occur here will be handled.)"
            n98 = Unbundle By Name(w254) -> ("Core.error"=w253:errorcluster)
            n99 = call <vilib>:"Add State(s) to Queue__jki_lib_state_machine.vi"("State(s) in (\"\")"=w258) -> ("States Out"=w257:string)  [unwired: 14 in]
          }
          frame "---------- Data ----------" {
            # "Do not put any code in this frame.\n(It is a separator no-op. You can make a copy of this frame to create a new Data frame)"
            n100 = call <vilib>:"Add State(s) to Queue__jki_lib_state_machine.vi"("State(s) in (\"\")"=w263) -> ("States Out"=w262:string)  [unwired: 14 in]
          }
          frame "Data: Initialize" {
            w265 = timestamp(0 s since 1904-01-01)  # switch time off
            w271 = refnum<class "Instrument.Oxford1820.lvclass"> refnum  # Instrument
            w275 = timestamp(0 s since 1904-01-01)  # LPF time
            w264 = timestamp(0 s since 1904-01-01)  # switch time on
            w277 = variant  # config
            w278 = ""  # Response
            w279 = T10 {"Current VI Reference"=refnum, "Close Panel on Exit?"=FALSE, "error"={"status"=FALSE, "code"=0, "source"=""}}  # Core
            # "do not delete - used by framework"
            # "Data names and types of shift register data are defined by this bundle."
            # "Initialize the shift-register data, here.\n(data names are defined by what you wire into the bundle function)"
            n101 = call <userlib>:"Read Instrument.vi"("error in (no error)"=w266, "Instrument UI in"=w267) -> ("error out"=w269:errorcluster, "Instrument"=w272:refnum<class "Instrument.lvclass">, "Instrument UI"=w273:refnum<class "Instrument UI.Oxford1820.lvclass">)  [unwired: 7 in]
            n102 = Get Date/Time In Seconds() -> (seconds since 1Jan1904=w276:timestamp)
            n103 = To More Specific Class(target class=w271, reference=w272) -> (specific class reference=w274:refnum<class "Instrument.Oxford1820.lvclass">)  [unwired: 1 in, 1 out]
            n104 = Variant To Data(error in=w269, type=w264, Variant=w276) -> (error out=w268:errorcluster)  [unwired: 1 out]
            n105 = Bundle("Core"=w279, "Instrument UI"=w273, "Instrument"=w274, "getAll"=T2 {"1820_IPS_Magnet_Field"=0.0, "1820_IPS_PS_Field"=0.0, "1820_IPS_Target_Field"=0.0, "1820_IPS_Target_Field_Rate"=0.0, "1820_IPS_Voltage"=0.0, "1820_IPS_Current"=0.0, "1820_IPS_Level_N2"=0.0, "1820_IPS_Level_He"=0.0, "1820_IPS_Magnet_Temperature"=0.0, "1820_IPS_Magnet_Temperature_R"=0.0, "1820_IPS_M1_Current"=0.0, "1820_IPS_M1_Voltage"=0.0, "1820_IPS_M2_Current"=0.0, "1820_IPS_M2_Voltage"=0.0, "1820_IPS_M3_Current"=0.0, "1820_IPS_M3_Voltage"=0.0, "1820_IPS_Status"="", "1820_IPS_Switch"="", "1820_ITC_Lambda_Temperature"=0.0, "1820_ITC_Lambda_Temperature_R"=0.0, "1820_ITC_Pressure"=0.0, "1820_ITC_Needle_Valve"=0.0}, "Response"=w278, "config"=w277, "switch time on"=w264, "switch time off"=w265, "LPF time"=w275) -> (w281:T8)  [unwired: 1 in]
            n106 = call <vilib>:"Add State(s) to Queue__jki_lib_state_machine.vi"("State(s) in (\"\")"=w283) -> ("States Out"=w282:string)  [unwired: 14 in]
          }
          frame "Data: Cleanup" {
            # "Cleanup any data and references, here.\n(this is called automatically, by the Macro: Exit)"
            n107 = Unbundle By Name(w285) -> ("Core.Current VI Reference"=w288:refnum<vi>)
            n108 = Close Reference(reference=w288, error in (no error)=w287) -> (error out=w286:errorcluster)
            n109 = call <vilib>:"Add State(s) to Queue__jki_lib_state_machine.vi"("State(s) in (\"\")"=w290) -> ("States Out"=w289:string)  [unwired: 14 in]
          }
          frame "---------- UI ----------" {
            # "Do not put any code in this frame.\n(It is a separator no-op. You can make a copy of this frame to create a new UI frame)"
            n110 = call <vilib>:"Add State(s) to Queue__jki_lib_state_machine.vi"("State(s) in (\"\")"=w295) -> ("States Out"=w294:string)  [unwired: 14 in]
          }
          frame "UI: Initialize" {
            # "size window to decoration box on front panel"
            # "Initialize the User Interface, here.\n(this is called automatically, by the Macro: Init)"
            n111 = property on="Window Minimize" class="Bool (strict)"("Value"=FALSE ("Window Maximize"), "Visible"=TRUE ("Window Maximize")) -> ()  [unwired: 2 in, 2 out]
            n112 = property on="Window Maximize" class="Bool (strict)"("Value"=FALSE ("Window Maximize"), "Visible"=FALSE ("Window Maximize")) -> ()  [unwired: 2 in, 2 out]
            n113 = call <userlib>:"Fit VI window to Largest Dec__ogtk.vi"("error in (no error)"=w306, "border spacing (2 px)"=0) -> ("error out"=w305:errorcluster)  [unwired: 4 in, 1 out]
            n114 = call <userlib>:"MGI Get Executable Version.vi"() -> ("Version"=w297:string)  [unwired: 7 in]
            n115 = Format Into String(format string="v%s", w297) -> (resulting string=→"version":string)  [unwired: 2 in, 1 out]
            n116 = local write "Level Graph"(cluster{timestamp[], dbl[]}[] [] ("XY Graph")) -> ()
            n117 = call <vilib>:"Add State(s) to Queue__jki_lib_state_machine.vi"("State(s) in (\"\")"=w310) -> ("States Out"=w309:string)  [unwired: 14 in]
          }
          frame "UI: Update Front Panel All" {
            n118 = Unbundle By Name(w315) -> ("getAll"=w318:T2)
            n119 = Unbundle By Name(w318) -> ("1820_IPS_Magnet_Field"=→"Field" →"Magnet Field Meter":dbl, "1820_IPS_PS_Field"=→"PSU Field":dbl, "1820_IPS_Target_Field"=→"Target Field (T)":dbl, "1820_IPS_Target_Field_Rate"=→"Target Rate (T/min)":dbl, "1820_IPS_Voltage"=→"Voltage" →"Voltage Meter":dbl, "1820_IPS_Current"=→"Current" →"Current Meter":dbl, "1820_IPS_Status"=w322:string, "1820_IPS_Switch"=w321:string, "1820_ITC_Lambda_Temperature"=→"Magnet T":dbl, "1820_ITC_Lambda_Temperature_R"=→"Magnet R":dbl, "1820_ITC_Pressure"=→"Pressure":dbl, "1820_ITC_Needle_Valve"=→"Needle Valve":dbl)  [unwired: 6 out]
            n120 = call "Action Status to Text.vi"("PSU Act Stat"=w322) -> ("Status:"=→"Magnet Status 3":string)
            n121 = call "Switch Status String to Boolean.vi"("String"=w321) -> ("Switch:"=w313:bool)
            n122 = Get Date/Time In Seconds() -> (seconds since 1Jan1904=w314:timestamp)
            n123 = call <userlib>:"Boolean Trigger__ogtk.vi"("Boolean Input"=w313) -> ("Rising Edge"=w312:bool, "Falling Edge"=w311:bool)  [unwired: 1 in]
            n124 = case shown="False" w313 {
              tunnel: [w336 w346] -> w316
              tunnel: w315 -> [w337 w345]
              tunnel: w314 -> [w335 w344]
              tunnel: w312 -> [_ w343]
              tunnel: w311 -> [w338 _]
              frame False {
                n125 = case shown="False" w338 {
                  tunnel: w337 -> [w339 w342]
                  tunnel: [w339 w341] -> w336
                  tunnel: w335 -> [_ w340]
                  frame False {
                  }
                  frame True {
                    n126 = Bundle By Name(cluster=w342, "switch time off"=w340) -> (w341:T8)
                  }
                }
              }
              frame True {
                n127 = case shown="True" w343 {
                  tunnel: [w347 w350] -> w346
                  tunnel: w345 -> [w347 w349]
                  tunnel: w344 -> [_ w348]
                  frame False {
                  }
                  frame True {
                    n128 = Bundle By Name(cluster=w349, "switch time on"=w348) -> (w350:T8)
                  }
                }
              }
            }
            n129 = local write "PS Heat"(w313) -> ()
            n130 = call <vilib>:"Add State(s) to Queue__jki_lib_state_machine.vi"("State(s) in (\"\")"=w334) -> ("States Out"=w333:string)  [unwired: 14 in]
          }
          frame "UI: Update Chart" {
            n131 = Unbundle By Name(w359) -> ("getAll"=w355:T2)
            n132 = Unbundle By Name(w355) -> ("1820_IPS_Level_N2"=w351:dbl, "1820_IPS_Level_He"=w352:dbl)  [unwired: 1 out]
            "He LEVEL" <- w352
            "He LVL" <- w352
            "He LVL Chart" <- w352
            "N2 LVL Chart" <- w351
            "N2 LVL" <- w351
            "N2 LEVEL" <- w351
            n133 = Build Array(w352, w351) -> (w356:dbl[])
            n134 = local read "Level Graph"() -> (w353:cluster{timestamp[], dbl[]}[])
            n135 = call "Time-Y Circ Buffer.vi"("buffer [1024]"=1024 ("y"), "Y in"=w356, "XY in"=w353) -> ("XY"=→"Level Graph":cluster{timestamp[], dbl[]}[])  [unwired: 8 in]
            n136 = call <vilib>:"Add State(s) to Queue__jki_lib_state_machine.vi"("State(s) in (\"\")"=w362) -> ("States Out"=w361:string)  [unwired: 14 in]
          }
          frame "UI: Update Front Panel Time" {
            n137 = Unbundle By Name(w380) -> ("switch time on"=w364:timestamp, "switch time off"=w365:timestamp, "LPF time"=w378:timestamp)
            n138 = local read "PS Heat"() -> (w366:bool)
            n139 = Get Date/Time In Seconds() -> (seconds since 1Jan1904=w371:timestamp)
            n140 = local read "LPF Power"() -> (w375:bool)
            n141 = local read "Target Rate (T/min)"() -> (w373:dbl)
            n142 = local read "Target Field (T)"() -> (w376:dbl)
            n143 = local read "PSU Field"() -> (w372:dbl)
            n144 = local read "Field"() -> (w374:dbl)
            n145 = To Double Precision Float(number=w371) -> (double precision float=→"System Time (HH:MM:SS)":dbl)
            n146 = Select(t=w364, s=w366, f=w365) -> (s? t:f=w363:timestamp)
            n147 = call "1820 LPF ON duration.vi"("Lambda"=w375, "LPF ON"=w378) -> ("LPF on (HH:MM:SS)"=→"LPF on":dbl)  [unwired: 9 in]
            n148 = call "1820 PS Heat duration.vi"("PS Heat"=TRUE, "time stamp"=w363) -> ("PS Heat on (HH:MM:SS)"=→"PS Heat on (HH:MM:SS)":dbl)  [unwired: 9 in]
            n149 = call "1820 Sweep ETA.vi"("Power Supply Field (T)"=w372, "Target Field Rate (T/min)"=w373, "Magnet Field (T)"=w374, "Target Field (T)"=w376) -> ("ETA timestamp"=w369:timestamp)  [unwired: 5 in, 2 out]
            n150 = To Double Precision Float(number=w369) -> (double precision float=→"ETA":dbl)
            n151 = call <vilib>:"Add State(s) to Queue__jki_lib_state_machine.vi"("State(s) in (\"\")"=w384) -> ("States Out"=w383:string)  [unwired: 14 in]
          }
          frame "UI: Status 2" {
            n152 = call <vilib>:"Add State(s) to Queue__jki_lib_state_machine.vi"("State(s) in (\"\")"=w390) -> ("States Out"=w389:string)  [unwired: 14 in]
            "Magnet Status 2" <- w385
          }
          frame "UI: Level Colors" {
            # "UI: Level Colors.\n(color level fill red/yello/green)"
            n153 = control-ref of="He LVL Chart"() -> (w392:refnum<vi>)
            n154 = call "Level Color.vi"("LVL Chart Refernce"=w392) -> ()  [unwired: 11 in]
            n155 = control-ref of="N2 LVL Chart"() -> (w391:refnum<vi>)
            n156 = call "Level Color.vi"("LVL Chart Refernce"=w391) -> ()  [unwired: 11 in]
            n157 = call <vilib>:"Add State(s) to Queue__jki_lib_state_machine.vi"("State(s) in (\"\")"=w397) -> ("States Out"=w396:string)  [unwired: 14 in]
          }
          frame "UI: Cursor Set" {
            # "Argument"
            # "Initialize the User Interface, here.\n(this is called automatically, by the Macro: Init)"
            n158 = disable-structure shown="Default" {
              disable-tunnel: w400 -> [w405 w408]
              disable-tunnel: [w405 w407] -> w399
              disable-tunnel: w398 -> [_ w406]
              frame condition #0 {
              }
              frame condition #1 (active) {
                n159 = case shown="\"Idle\", Default" w406 {
                  tunnel: w408 -> [w410 w412]
                  tunnel: [w409 w411] -> w407
                  frame "Idle", Default {
                    n160 = call <vilib>:"Unset Busy.vi"("error in (no error)"=w410) -> ("error out"=w409:errorcluster)  [unwired: 10 in]
                  }
                  frame "Busy" {
                    n161 = call <vilib>:"Set Busy.vi"("error in (no error)"=w412) -> ("error out"=w411:errorcluster)  [unwired: 9 in, 1 out]
                  }
                }
              }
            }
            n162 = call <vilib>:"Add State(s) to Queue__jki_lib_state_machine.vi"("State(s) in (\"\")"=w404) -> ("States Out"=w403:string)  [unwired: 14 in]
          }
          frame "UI: Front Panel State" {
            # "Argument"
            # "Set Front Panel Open or Closed\n(Usage: \"UI: Front Panel State >> Open|Close\")"
            n163 = Unbundle By Name(w416) -> ("Core.Current VI Reference"=w415:refnum<vi>)
            n164 = disable-structure shown="Default" {
              disable-tunnel: w418 -> [w424 w447]
              disable-tunnel: [w423 w447] -> w417
              disable-tunnel: w415 -> [w422 _]
              disable-tunnel: w414 -> [w421 _]
              frame condition #0 (active) {
                n165 = case shown="\"Open\", Default" w421 {
                  tunnel: w424 -> [w428 w441]
                  tunnel: [w430 w442] -> w423
                  tunnel: w422 -> [w429 w439]
                  frame "Open", Default {
                    n166 = property class="VI"(reference=w429, error in=w428) -> (reference out=w426:refnum<vi>, error out=w427:errorcluster, "FP.State"=w425:T4)
                    n167 = case shown="\"Closed\"" w425 {
                      tunnel: [w433 w436] -> w430
                      tunnel: w427 -> [w432 w436]
                      tunnel: w426 -> [w431 _]
                      frame "Closed" {
                        n168 = invoke class="VI" method="FP.Open"(reference=w431, error in=w432, "Activate"=TRUE, "State"=T4."Standard") -> (error out=w433:errorcluster)  [unwired: 1 in, 4 out]
                      }
                      frame Default {
                      }
                    }
                  }
                  frame "Close" {
                    n169 = property class="VI"(reference=w439, error in=w441) -> (reference out=w438:refnum<vi>, error out=w440:errorcluster, "FP.State"=w437:T4)
                    n170 = case shown="Default" w437 {
                      tunnel: [w443 w446] -> w442
                      tunnel: w440 -> [w443 w445]
                      tunnel: w438 -> [_ w444]
                      frame "Invalid", "Closed" {
                      }
                      frame Default {
                        n171 = invoke class="VI" method="FP.Close"(reference=w444, error in=w445) -> (error out=w446:errorcluster)  [unwired: 1 in, 2 out]
                      }
                    }
                  }
                }
              }
              frame condition #1 {
              }
            }
            n172 = call <vilib>:"Add State(s) to Queue__jki_lib_state_machine.vi"("State(s) in (\"\")"=w420) -> ("States Out"=w419:string)  [unwired: 14 in]
          }
          frame "UI: Minimize" {
            # "Do not put any code in this frame.\n(It is a separator no-op. You can make a copy of this frame to create a new UI frame)"
            n173 = Unbundle By Name(w453) -> ("Core.Current VI Reference"=w452:refnum<vi>)
            n174 = property class="VI"(reference=w452, error in=w449) -> (reference out=w451:refnum<vi>, error out=w450:errorcluster, "Front Panel.PanelBounds"=w457:T11)
            n175 = case shown="\"Min\", Default" w455 {
              tunnel: w457 -> [w460 w468]
              tunnel: [w467 w475] -> w456
              frame "Min", Default {
                n176 = Unbundle By Name(w460) -> ("Left"=w466:i16, "Top"=w464:i16)
                n177 = Add(x=i16 776 ("x 6"), y=w466) -> (x+y=w465:i16)
                n178 = Add(x=w464, y=i16 184 ("x 5")) -> (x+y=w463:i16)
                n179 = Bundle By Name(cluster=w460, "Right"=w465, "Bottom"=w463) -> (w467:T11)
              }
              frame "Max" {
                n180 = Unbundle By Name(w468) -> ("Left"=w474:i16, "Top"=w472:i16)
                n181 = Add(x=i16 1168 ("x 8"), y=w474) -> (x+y=w473:i16)
                n182 = Add(x=w472, y=i16 584 ("x 7")) -> (x+y=w471:i16)
                n183 = Bundle By Name(cluster=w468, "Right"=w473, "Bottom"=w471) -> (w475:T11)
              }
            }
            n184 = property class="VI"(reference=w451, error in=w450, "Front Panel.PanelBounds"=w456) -> (error out=w448:errorcluster)  [unwired: 1 out]
            n185 = call <vilib>:"Add State(s) to Queue__jki_lib_state_machine.vi"("State(s) in (\"\")"=w454) -> ("States Out"=w459:string)  [unwired: 14 in]
          }
          frame "---------- Macro ----------" {
            # "Do not put any code in this frame.\n(It is a separator no-op. You can make a copy of this frame to create a new Macro frame)"
            n186 = call <vilib>:"Add State(s) to Queue__jki_lib_state_machine.vi"("State(s) in (\"\")"=w480) -> ("States Out"=w479:string)  [unwired: 14 in]
          }
          frame "Macro: Initialize" {
            w483 = "UI: Initialize\nUI: Front Panel State >> Open\nAction: Open\nUI: Status 2 >> ..."  # UI: Initialize UI: Front Panel State >> Open Action: Open UI: Status 2 >> ...
            # "Initialization Macro\n(This is called once, when the VI starts)"
            n187 = call <vilib>:"Add State(s) to Queue__jki_lib_state_machine.vi"("State(s) in Front (\"\")"="Data: Initialize\nInitialize Core Data\nEvents: Register", "State(s) in (\"\")"="Process: Sync", "State(s) at Back (\"\")"=w483) -> ("States Out"=w482:string)  [unwired: 12 in]
            n188 = call <vilib>:"Add State(s) to Queue__jki_lib_state_machine.vi"("State(s) in Front (\"\")"=w482, "State(s) in (\"\")"=w489) -> ("States Out"=w488:string)  [unwired: 13 in]
          }
          frame "Macro: Exit" {
            # "Exit Macro\n(This is called once, when the VI exits)"
            n189 = Unbundle By Name(w494) -> ("Core.Close Panel on Exit?"=w500:bool)
            n190 = Select(t="UI: Front Panel State >> Close", s=w500, f="") -> (s? t:f=w497:string)
            n191 = call <vilib>:"Add State(s) to Queue__jki_lib_state_machine.vi"("State(s) in Front (\"\")"="Data: Cleanup\nEvents: Unregister\nProcess: Self Terminate", "State(s) in (\"\")"="Process: Sync", "State(s) at Back (\"\")"="Exit") -> ("States Out"=w491:string)  [unwired: 12 in]
            n192 = call <vilib>:"Add State(s) to Queue__jki_lib_state_machine.vi"("State(s) in (\"\")"=w497, "State(s) at Back (\"\")"=w491) -> ("States Out"=w496:string)  [unwired: 13 in]
            n193 = call <vilib>:"Add State(s) to Queue__jki_lib_state_machine.vi"("State(s) in Front (\"\")"=w496, "State(s) in (\"\")"=w503) -> ("States Out"=w502:string)  [unwired: 13 in]
          }
          frame "---------- Process ----------" {
            # "Template Separator\n(You can make a copy of, or modify, this frame)"
            n194 = call <vilib>:"Add State(s) to Queue__jki_lib_state_machine.vi"("State(s) in (\"\")"=w508) -> ("States Out"=w507:string)  [unwired: 14 in]
          }
          frame "Process: Sync" {
            n195 = Unbundle By Name(w516) -> ("Instrument UI"=w512:refnum<class "Instrument UI.Oxford1820.lvclass">)
            n196 = call <vilib>:"WaitOnProcessSync.vi"("error in (no error)"=w511, "SMO"=w512) -> ("error out"=w510:errorcluster, "Don't run?"=w515:bool)  [unwired: 7 in, 1 out]
            n197 = Select(t="Data: Cleanup\nEvents: Unregister\nExit", s=w515, f="") -> (s? t:f=w509:string)
            n198 = call <vilib>:"Add State(s) to Queue__jki_lib_state_machine.vi"("State(s) in Front (\"\")"=w509, "State(s) in (\"\")"=w519) -> ("States Out"=w518:string)  [unwired: 13 in]
          }
          frame "Process: Self Terminate" {
            n199 = Unbundle By Name(w521) -> ("Instrument UI"=w520:refnum<class "Instrument UI.Oxford1820.lvclass">)
            n200 = call <vilib>:"SelfTerminate.vi"("error in (no error)"=w523, "SMO in"=w520) -> ("error out"=w522:errorcluster)  [unwired: 8 in, 1 out]
            n201 = call <vilib>:"Add State(s) to Queue__jki_lib_state_machine.vi"("State(s) in (\"\")"=w526) -> ("States Out"=w525:string)  [unwired: 14 in]
          }
          frame "---------- Events ----------" {
            # "Template Separator\n(You can make a copy of, or modify, this frame)"
            n202 = call <vilib>:"Add State(s) to Queue__jki_lib_state_machine.vi"("State(s) in (\"\")"=w531) -> ("States Out"=w530:string)  [unwired: 14 in]
          }
          frame "Events: Register" {
            # "Expand to add\nmore events"
            # "Base Class Protected Events"
            n203 = Unbundle By Name(w545) -> ("Instrument UI"=w540:refnum<class "Instrument UI.Oxford1820.lvclass">, "Instrument"=w538:refnum<class "Instrument.Oxford1820.lvclass">)
            n204 = call <vilib>:"GetProtectedEvents.vi"("SMO"=w540) -> ("error out"=w541:errorcluster, "SMO Protected Events"=w543:T12)  [unwired: 8 in, 1 out]
            n205 = call <userlib>:"Instrument.GetPublicEvents.vi"("Instrument"=w538) -> ("error out"=w539:errorcluster, "Instrument Public Events"=w537:T13, "Instrument out"=w536:refnum<class "Instrument.Oxford1820.lvclass">)  [unwired: 8 in]
            n206 = call "Instrument.Oxford1820.GetPublicEvents.vi"("Instrument.Oxford1820 in"=w536) -> ("error out"=w534:errorcluster, "OI1820 Public Events"=w535:T14)  [unwired: 8 in, 1 out]
            n207 = register-events(w543, w537, w535) -> (reference out=w544:refnum<event-registration>, error out=w532:errorcluster)  [unwired: 2 in]
            n208 = Merge Errors(w532, w534, w539, w541, w533) -> (w542:errorcluster)
            n209 = call <vilib>:"Add State(s) to Queue__jki_lib_state_machine.vi"("State(s) in (\"\")"=w547) -> ("States Out"=w546:string)  [unwired: 14 in]
          }
          frame "Events: Unregister" {
            n210 = Unregister For Events(event registration refnum=w550, error in=w549) -> (error out=w548:errorcluster)
            n211 = call <vilib>:"Add State(s) to Queue__jki_lib_state_machine.vi"("State(s) in (\"\")"=w553) -> ("States Out"=w552:string)  [unwired: 14 in]
          }
          frame "---------- Action ----------" {
            n212 = Unbundle By Name(w556) -> ("Instrument UI"=w554:refnum<class "Instrument UI.Oxford1820.lvclass">)
            n213 = Bundle By Name(cluster=w556, "Instrument UI"=w554) -> (w555:T8)
            n214 = call <vilib>:"Add State(s) to Queue__jki_lib_state_machine.vi"("State(s) in (\"\")"=w560) -> ("States Out"=w559:string)  [unwired: 14 in]
          }
          frame "Action: Notify UI Closed" {
            # "Notify that the UI has been closed"
            n215 = Unbundle By Name(w561) -> ("Instrument UI"=w564:refnum<class "Instrument UI.Oxford1820.lvclass">)
            n216 = call <vilib>:"Hide.vi"("error in (no error)"=w563, "SMO.UI"=w564) -> ("error out"=w562:errorcluster)  [unwired: 8 in, 1 out]
            n217 = call <vilib>:"Add State(s) to Queue__jki_lib_state_machine.vi"("State(s) in (\"\")"=w567) -> ("States Out"=w566:string)  [unwired: 14 in]
          }
          frame "Action: Open" {
            n218 = Unbundle By Name(w574) -> ("Instrument"=w571:refnum<class "Instrument.Oxford1820.lvclass">)
            n219 = call <userlib>:"Write Client Type.vi"("error in (no error)"=w569, "Client Type [Remote]"=Client_Type--Enum."Local", "Instrument in"=w571) -> ("error out"=w572:errorcluster, "Instrument out"=w570:refnum<class "Instrument.Oxford1820.lvclass">)  [unwired: 7 in]
            n220 = Bundle By Name(cluster=w574, "Instrument"=w570) -> (w573:T8)
            n221 = call <vilib>:"Add State(s) to Queue__jki_lib_state_machine.vi"("State(s) in (\"\")"=w577) -> ("States Out"=w576:string)  [unwired: 14 in]
          }
          frame "Action: get All" {
            n222 = Unbundle By Name(w580) -> ("Instrument"=w583:refnum<class "Instrument.Oxford1820.lvclass">)
            n223 = call "Instrument.Oxford1820.Get All.vi"("error in (no error)"=w579, "Instrument.Oxford1820 in"=w583) -> ("error out"=w582:errorcluster, "getAll"=w578:T2, "Instrument.Oxford1820 out"=w581:refnum<class "Instrument.Oxford1820.lvclass">)  [unwired: 7 in]
            n224 = Bundle By Name(cluster=w580, "Instrument"=w581, "getAll"=w578) -> (w584:T8)
            n225 = call <vilib>:"Add State(s) to Queue__jki_lib_state_machine.vi"("State(s) in (\"\")"=w587) -> ("States Out"=w586:string)  [unwired: 14 in]
          }
          frame "Action: Hold" {
            n226 = Unbundle By Name(w588) -> ("Instrument"=w592:refnum<class "Instrument.Oxford1820.lvclass">)
            n227 = call "Hold.vi"("error in (no error)"=w591, "Instrument.1820 in"=w592) -> ("error out"=w593:errorcluster, "Instrument.1820 in"=w589:refnum<class "Instrument.Oxford1820.lvclass">)  [unwired: 7 in, 1 out]
            n228 = Bundle By Name(cluster=w588, "Instrument"=w589) -> (w590:T8)
            n229 = call <vilib>:"Add State(s) to Queue__jki_lib_state_machine.vi"("State(s) in (\"\")"=w596) -> ("States Out"=w595:string)  [unwired: 14 in]
          }
          frame "Action: Abort Sequence" {
            n230 = Unbundle By Name(w597) -> ("Instrument"=w600:refnum<class "Instrument.Oxford1820.lvclass">)
            n231 = call "Instrument.Oxford1820.AbortSequence.vi"("error in (no error)"=w599, "Instrument.Oxford1820"=w600) -> ("error out"=w598:errorcluster)  [unwired: 8 in, 1 out]
            n232 = call <vilib>:"Add State(s) to Queue__jki_lib_state_machine.vi"("State(s) in (\"\")"=w603) -> ("States Out"=w602:string)  [unwired: 14 in]
          }
          frame "Action: To Zero" {
            n233 = Unbundle By Name(w606) -> ("Instrument"=w608:refnum<class "Instrument.Oxford1820.lvclass">)
            n234 = call "Ramp to Zero.vi"("error in (no error)"=w607, "Instrument.1820 in"=w608) -> ("error out"=w609:errorcluster, "Instrument.1820 in"=w604:refnum<class "Instrument.Oxford1820.lvclass">)  [unwired: 8 in]
            n235 = Bundle By Name(cluster=w606, "Instrument"=w604) -> (w605:T8)
            n236 = call <vilib>:"Add State(s) to Queue__jki_lib_state_machine.vi"("State(s) in (\"\")"=w612) -> ("States Out"=w611:string)  [unwired: 14 in]
          }
          frame "Action: To Set" {
            n237 = Unbundle By Name(w615) -> ("Instrument"=w617:refnum<class "Instrument.Oxford1820.lvclass">)
            n238 = call "Ramp to Set.vi"("error in (no error)"=w616, "Instrument.1820 in"=w617) -> ("error out"=w618:errorcluster, "Instrument.1820 in"=w613:refnum<class "Instrument.Oxford1820.lvclass">)  [unwired: 7 in, 1 out]
            n239 = Bundle By Name(cluster=w615, "Instrument"=w613) -> (w614:T8)
            n240 = call <vilib>:"Add State(s) to Queue__jki_lib_state_machine.vi"("State(s) in (\"\")"=w621) -> ("States Out"=w620:string)  [unwired: 14 in]
          }
          frame "Action: Clamp" {
            n241 = Unbundle By Name(w624) -> ("Instrument"=w626:refnum<class "Instrument.Oxford1820.lvclass">)
            n242 = call "Clamp.vi"("error in (no error)"=w625, "Instrument.1820 in"=w626) -> ("error out"=w627:errorcluster, "Instrument.1820 in"=w622:refnum<class "Instrument.Oxford1820.lvclass">)  [unwired: 7 in, 1 out]
            n243 = Bundle By Name(cluster=w624, "Instrument"=w622) -> (w623:T8)
            n244 = call <vilib>:"Add State(s) to Queue__jki_lib_state_machine.vi"("State(s) in (\"\")"=w630) -> ("States Out"=w629:string)  [unwired: 14 in]
          }
          frame "Action: Fill" {
            n245 = Unbundle By Name(w635) -> ("Instrument"=w640:refnum<class "Instrument.Oxford1820.lvclass">)
            n246 = Select(t=T6 "OFF" ("Fill Mode"), s="Fast/Slow Fill", f=T6 "ON" ("Fill Mode")) -> (s? t:f=w636:T6)
            n247 = call "Set Fill Mode.vi"("error in (no error)"=w639, "Fill Mode"=w636, "Instrument.1820 in"=w640) -> ("error out"=w638:errorcluster, "Instrument.1820 in"=w633:refnum<class "Instrument.Oxford1820.lvclass">)  [unwired: 6 in, 1 out]
            n248 = Bundle By Name(cluster=w635, "Instrument"=w633) -> (w634:T8)
            n249 = call <vilib>:"Add State(s) to Queue__jki_lib_state_machine.vi"("State(s) in (\"\")"=w643) -> ("States Out"=w642:string)  [unwired: 14 in]
          }
          frame "Action: LPF" {
            n250 = Unbundle By Name(w648) -> ("Instrument"=w654:refnum<class "Instrument.Oxford1820.lvclass">)
            n251 = Select(t=T1 "ON" ("LPF State"), s="LPF Power", f=T1 "OFF" ("LPF State")) -> (s? t:f=w651:T1)
            n252 = call "Set LPF State.vi"("error in (no error)"=w653, "LPF State"=w651, "Instrument.1820 in"=w654) -> ("error out"=w652:errorcluster, "Instrument.1820 in"=w645:refnum<class "Instrument.Oxford1820.lvclass">)  [unwired: 6 in, 1 out]
            n253 = Get Date/Time In Seconds() -> (seconds since 1Jan1904=w647:timestamp)
            n254 = Bundle By Name(cluster=w648, "LPF time"=w647, "Instrument"=w645) -> (w646:T8)
            n255 = call <vilib>:"Add State(s) to Queue__jki_lib_state_machine.vi"("State(s) in (\"\")"=w657) -> ("States Out"=w656:string)  [unwired: 14 in]
          }
          frame "Action: Needle Valve" {
            # "2=open"
            # "1=closed"
            n256 = Unbundle By Name(w661) -> ("Instrument"=w669:refnum<class "Instrument.Oxford1820.lvclass">)
            n257 = Build Array("Close Needle Valve", "Open Needle Valve") -> (w667:bool[])
            n258 = Boolean Array To Number(Boolean array=w667) -> (number=w665:u32)
            n259 = case shown="1, Default" w665 {
              tunnel: [0.0 ("Needle Valve (%)") "Open Target"] -> w664
              frame 1, Default {
              }
              frame 2 {
              }
            }
            n260 = call "Set Needle Valve.vi"("error in (no error)"=w668, "Needle Valve (%)"=w664, "Instrument.1820 in"=w669) -> ("error out"=w663:errorcluster, "Instrument.1820 in"=w659:refnum<class "Instrument.Oxford1820.lvclass">)  [unwired: 6 in, 1 out]
            n261 = flat-sequence {
              tunnel: [w673] -> w662
              tunnel: w663 -> [w673]
              frame #0 {
                n262 = local write "Close Needle Valve"(FALSE ("Close Needle Valve")) -> ()
                n263 = local write "Open Needle Valve"(FALSE ("Open Needle Valve")) -> ()
              }
            }
            n264 = Bundle By Name(cluster=w661, "Instrument"=w659) -> (w660:T8)
            n265 = call <vilib>:"Add State(s) to Queue__jki_lib_state_machine.vi"("State(s) in (\"\")"=w672) -> ("States Out"=w671:string)  [unwired: 14 in]
          }
          frame "Action: PS Heat" {
            n266 = Unbundle By Name(w679) -> ("Instrument"=w681:refnum<class "Instrument.Oxford1820.lvclass">)
            n267 = call "Set Switch Heater.vi"("error in (no error)"=w685, "Switch Heater"=w680, "Instrument.1820 in"=w681) -> ("error out"=w684:errorcluster, "Instrument.1820 in"=w678:refnum<class "Instrument.Oxford1820.lvclass">)  [unwired: 6 in, 1 out]
            n268 = Get Date/Time In Seconds() -> (seconds since 1Jan1904=w683:timestamp)
            n269 = Bundle By Name(cluster=w679, "switch time on"=w683, "Instrument"=w678) -> (w682:T8)
            n270 = call <vilib>:"Add State(s) to Queue__jki_lib_state_machine.vi"("State(s) in (\"\")"=w688) -> ("States Out"=w687:string)  [unwired: 14 in]
          }
          frame "Action: Send to IPS" {
            n271 = Unbundle By Name(w691) -> ("Instrument"=w696:refnum<class "Instrument.Oxford1820.lvclass">)
            n272 = call "Set Target.vi"("error in (no error)"=w695, "Target Rate (T/min)"="Target Rate (T/min)", "Target Field (T)"="Target Field (T)", "Instrument.1820 in"=w696) -> ("error out"=w694:errorcluster, "Instrument.1820 in"=w689:refnum<class "Instrument.Oxford1820.lvclass">)  [unwired: 5 in, 1 out]
            n273 = Bundle By Name(cluster=w691, "Instrument"=w689) -> (w690:T8)
            n274 = call <vilib>:"Add State(s) to Queue__jki_lib_state_machine.vi"("State(s) in (\"\")"=w699) -> ("States Out"=w698:string)  [unwired: 14 in]
          }
        }
      }
    }
    frame Error {
    }
  }
  n275 = call-parent "Process.vi"("error in"=w6, "Instrument UI in"=w5) -> ("error out"=w3:errorcluster, "Instrument UI out"=→"Oxford1820 UI out":refnum<class "Instrument UI.Oxford1820.lvclass">)  [unwired: 8 in]
  n276 = Merge Errors(w3, w2) -> (→"error out":errorcluster)
